vi "FibonacciSequence-ShiftRegistersDemo.vi"() -> ()   [LabVIEW 2018]
panel:
  in  "?":bool
  in  "Terms to Calculate":dbl=10.0 min=2.0 max=30.0 step=1.0 format="%#_2g"
  out "Fibonacci Sequence:":string
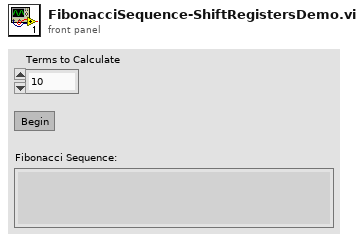
[diagram p1: front panel]
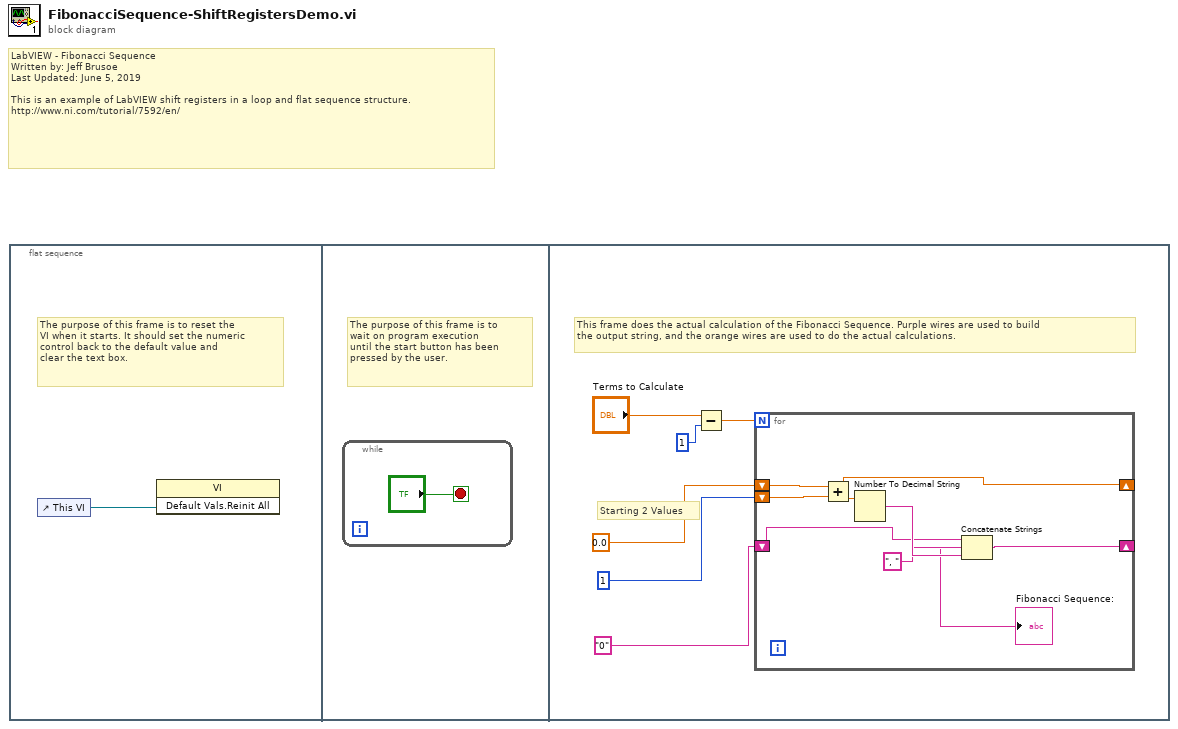
[diagram p0: block diagram]
diagram:
  # "LabVIEW - Fibonacci Sequence \nWritten by: Jeff Brusoe\nLast Updated: June 5, 2019\n\nThis is an example of LabVIEW shift registers in a loop and flat sequence structure.\nhttp://www.ni.com/tutorial/7592/en/"
  n1 = flat-sequence {
    frame #0 {
      # "The purpose of this frame is to reset the\nVI when it starts. It should set the numeric\ncontrol back to the default value and \nclear the text box."
      n2 = control-ref of="This VI"() -> (w1:refnum<vi>)
      n3 = invoke class="VI" method="Default Vals.Reinit All"(reference=w1) -> ()  [unwired: 2 in, 3 out]
    }
    frame #1 {
      # "The purpose of this frame is to\nwait on program execution\nuntil the start button has been\npressed by the user."
      n4 = while {
        stop <- "?" stop-if-true
      }
    }
    frame #2 {
      # "This frame does the actual calculation of the Fibonacci Sequence. Purple wires are used to build\nthe output string, and the orange wires are used to do the actual calculations."
      # "Starting 2 Values"
      n5 = Subtract(x="Terms to Calculate", y=1) -> (x-y=w8:dbl)
      n6 = for {
        N: w8 -> [_]
        shift-right: [w13] -> _
        shift-left: 0.0 -> [w15]
        shift-left: 1 -> [w14]
        shift-right: [w9] -> _
        shift-left: "0" -> [w10]
        n7 = Add(x=w15, y=w14) -> (x+y=w13:dbl)
        n8 = Number To Decimal String(number=w13) -> (decimal integer string=w12:string)  [unwired: 1 in]
        n9 = Concatenate Strings(w10, ", ", w12) -> (w9:string)
        "Fibonacci Sequence:" <- w9
      }
    }
  }
